vi "Adjust Times.vi"(8 "error in":errorcluster, 11 "Times":string[](array[string])) -> (0 "error out":errorcluster, 1 "Event Times":dbl[](array[numeric]), 2 "End Times":dbl[](array[numeric]), 3 "Start Times":dbl[](array[numeric]))   [LabVIEW 2021]
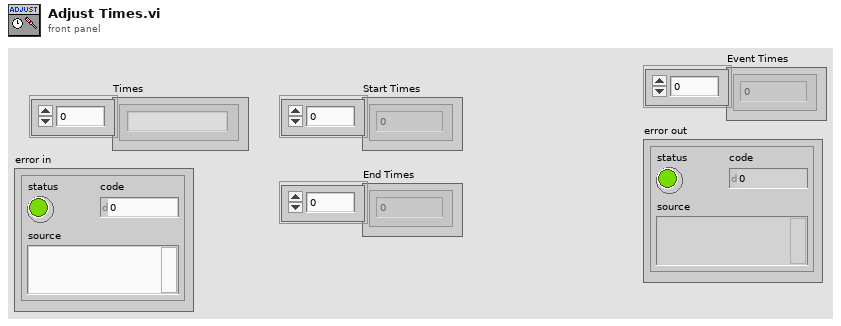
[diagram p1: front panel]
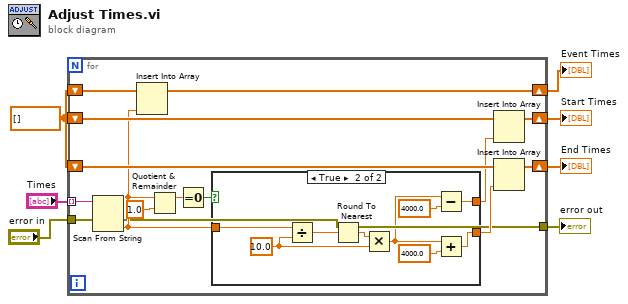
[diagram p0: block diagram]
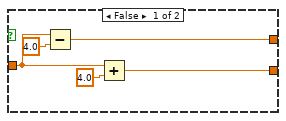
[diagram p2: hidden frame]
diagram:
  w4 = dbl[] []
  n1 = for {
    tunnel: "Times" -> [w16] mode=indexing
    shift-right: [w21] -> w6
    shift-left: w4 -> [w22]
    shift-right: [w19] -> w7
    shift-left: w4 -> [w20]
    shift-right: [w11] -> w3
    shift-left: w4 -> [w12]
    tunnel: [w9] -> w1
    tunnel: "error in" -> [w8]
    n2 = Scan From String(input string=w16, error in=w8) -> (error out=w9:errorcluster, output 1=w10:dbl)  [unwired: 3 in, 2 out]
    n3 = Insert Into Array(array=w12, new element=w10) -> (w11:dbl[])  [unwired: 1 in]
    n4 = Quotient & Remainder(x=w10, y=1.0) -> (x-y*floor(x/y)=w14:dbl)  [unwired: 1 out]
    n5 = Equal To 0?(x=w14) -> (x = 0?=w13:bool)
    n6 = case shown="True" w13 {
      tunnel: w10 -> [w26 w31]
      tunnel: [w23 w29] -> w18
      tunnel: [w24 w28] -> w17
      frame False {
        n7 = Subtract(x=w26, y=4.0) -> (x-y=w24:dbl)
        n8 = Add(x=w26, y=4.0) -> (x+y=w23:dbl)
      }
      frame True {
        w33 = 10.0 ("y")
        n9 = Divide(x=w31, y=w33) -> (x/y=w34:dbl)
        n10 = Round To Nearest(number=w34) -> (nearest integer value=w35:dbl)
        n11 = Multiply(x=w35, y=w33) -> (x*y=w36:dbl)
        n12 = Subtract(x=w36, y=4000.0) -> (x-y=w28:dbl)
        n13 = Add(x=w36, y=4000.0) -> (x+y=w29:dbl)
      }
    }
    n14 = Insert Into Array(array=w22, new element=w17) -> (w21:dbl[])  [unwired: 1 in]
    n15 = Insert Into Array(array=w20, new element=w18) -> (w19:dbl[])  [unwired: 1 in]
  }
  "End Times" <- w7
  "Start Times" <- w6
  "Event Times" <- w3
  "error out" <- w1
